vi "Configure Math (Unary Operation).vi"(0 "VISA resource name":refnum<visa-resource-name>, 1 "Enable Math Channel (T:Enable)":bool=TRUE, 2 "# of Averages (16)":i32=16, 3 "FFTWindow (0:Rectangular)":u16(ring) items=["Rectangular", "Hanning", "FlatTop"], 5 "Math Channel (5: Function 1)":i32(ring)=5 items=["Function 1"=5, "Function 2"=6, "Function 3"=7, "Function 4"=8], 7 "Math Operand (1: Channel 1)":i32(ring)=1 items=["Channel 1"=1, "Channel 2"=2, "Channel 3"=3, "Channel 4"=4, "Function 1"=5, "Function 2"=6, "Function 3"=7, "Function 4"=8, "Memory 1"=9, "Memory 2"=10, "Memory 3"=11, "Memory 4"=12], 9 "Math Operation (0: Average)":u16(ring) items=["Average", "Differentiate", "FFT Magnitude", "FFT Phase", "High Pass Filter", "Integrate", "Invert", "Low Pass Filter", "Magnify", "Max", "Min", "Smooth"], 11 "error in (no error)":errorcluster, 12 "Bandwidth (350E6)":dbl=350000000.0, 13 "Smoothing Points (5)":i32=5) -> (4 "VISA resource name out":refnum<visa-resource-name>, 15 "error out":errorcluster)   [LabVIEW 2009, in "Agilent 8000 Series.lvlib"]
doc: "Creates a mathematical expression with one operand."
uses:
  Agilent 8000 Series.lvlib
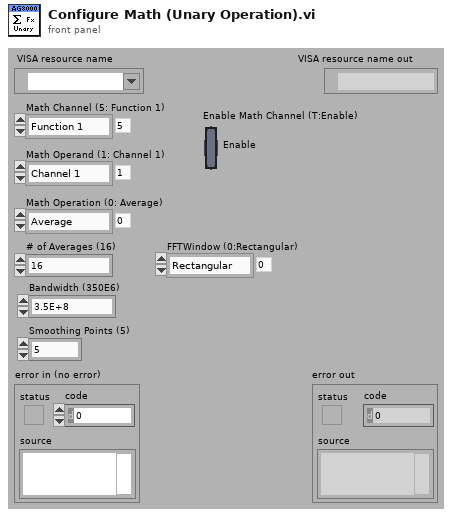
[diagram p1: front panel]
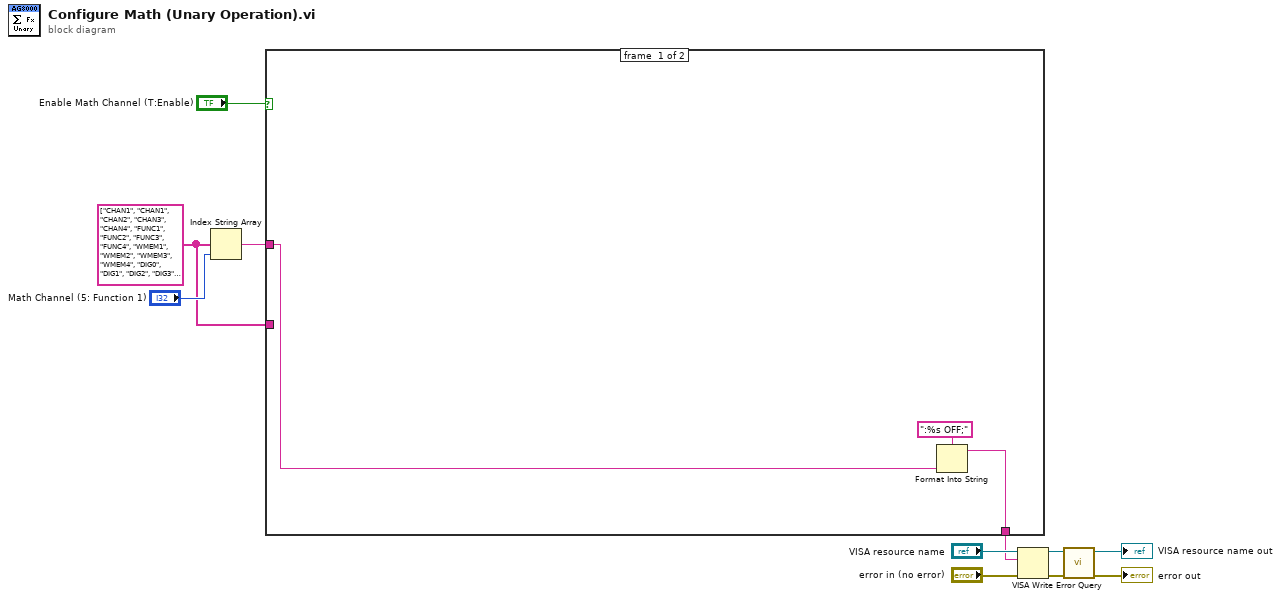
[diagram p0: block diagram]
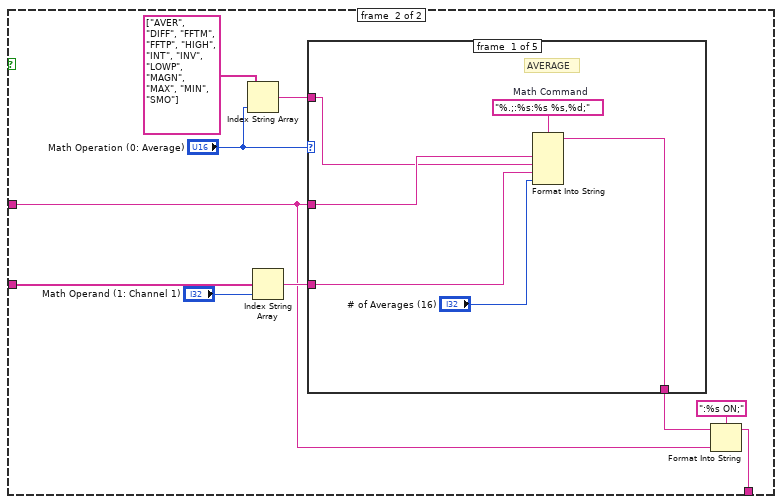
[diagram p2: hidden frame]
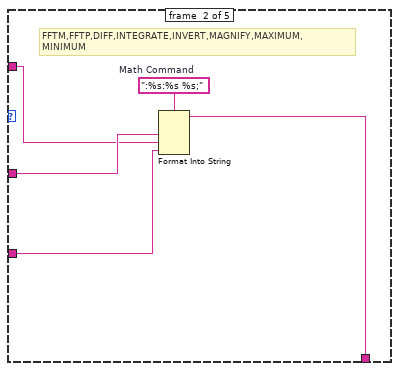
[diagram p3: hidden frame]
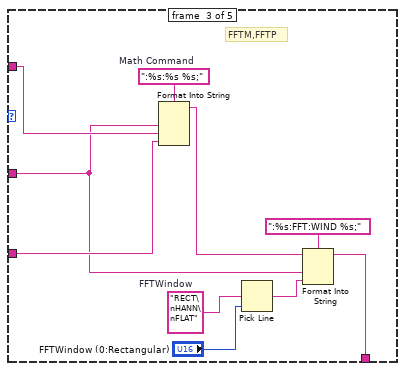
[diagram p4: hidden frame]
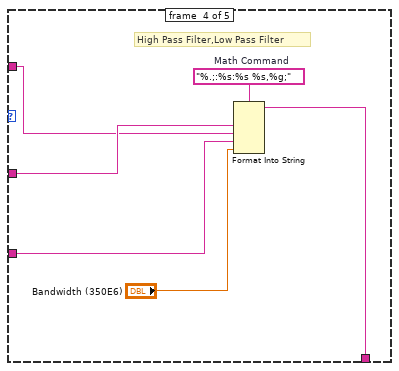
[diagram p5: hidden frame]
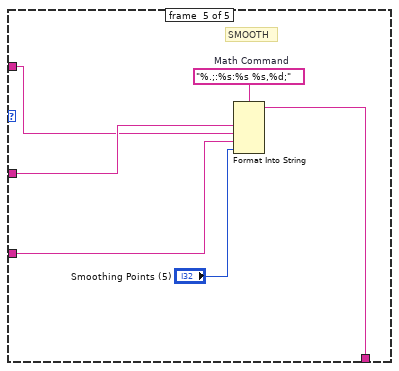
[diagram p6: hidden frame]
diagram:
  w3 = string[] ["CHAN1", "CHAN1", "CHAN2", "CHAN3", "CHAN4", "FUNC1", "FUNC2", "FUNC3", "FUNC4", "WMEM1", "WMEM2", "WMEM3", "WMEM4", "DIG0", "DIG1", "DIG2", "DIG3", "DIG4", "DIG5", "DIG6", "DIG7", "DIG8", "DIG9", "DIG10", "DIG11", "DIG12", "DIG13", "DIG14", "DIG15", "AUX", "LINE"]
  n1 = Index String Array(1:"Math Channel (5: Function 1)", 2:w3) -> (0:w4:string)  [unwired: 1 in]
  n2 = case shown="True" "Enable Math Channel (T:Enable)" {
    tunnel: w4 -> [w13 w16]
    tunnel: w3 -> [_ w20]
    tunnel: [w12 w15] -> w1
    frame #0 {
      n3 = Format Into String(format string=":%s OFF;", w13) -> (resulting string=w12:string)  [unwired: 2 in, 1 out]
    }
    frame #1 {
      n4 = Index String Array(1:"Math Operation (0: Average)", 2:string[] ["AVER", "DIFF", "FFTM", "FFTP", "HIGH", "INT", "INV", "LOWP", "MAGN", "MAX", "MIN", "SMO"]) -> (0:w22:string)  [unwired: 1 in]
      n5 = Index String Array(1:"Math Operand (1: Channel 1)", 2:w20) -> (0:w19:string)  [unwired: 1 in]
      n6 = case shown="11" "Math Operation (0: Average)" {
        tunnel: w16 -> [w30 w35 w37 w51 w57]
        tunnel: w22 -> [w29 w34 w45 w50 w56]
        tunnel: w19 -> [w28 w33 w44 w49 w55]
        tunnel: [w25 w31 w36 w46 w52] -> w18
        frame #0 {
          w27 = "%.;:%s:%s %s,%d;"  # Math Command
          # "AVERAGE"
          n7 = Format Into String(format string=w27, w30, w29, w28, "# of Averages (16)") -> (resulting string=w25:string)  [unwired: 2 in, 1 out]
        }
        frame #1 {
          w32 = ":%s:%s %s;"  # Math Command
          # "FFTM,FFTP,DIFF,INTEGRATE,INVERT,MAGNIFY,MAXIMUM,\nMINIMUM"
          n8 = Format Into String(format string=w32, w35, w34, w33) -> (resulting string=w31:string)  [unwired: 2 in, 1 out]
        }
        frame #2 {
          w42 = "RECT\nHANN\nFLAT"  # FFTWindow
          w43 = ":%s:%s %s;"  # Math Command
          # "FFTM,FFTP"
          n9 = Format Into String(format string=w43, w37, w45, w44) -> (resulting string=w39:string)  [unwired: 2 in, 1 out]
          n10 = Pick Line(multi-line string=w42, line index="FFTWindow (0:Rectangular)") -> (output string=w38:string)  [unwired: 1 in]
          n11 = Format Into String(format string=":%s:FFT:WIND %s;", initial string=w39, w37, w38) -> (resulting string=w36:string)  [unwired: 1 in, 1 out]
        }
        frame #3 {
          w48 = "%.;:%s:%s %s,%g;"  # Math Command
          # "High Pass Filter,Low Pass Filter"
          n12 = Format Into String(format string=w48, w51, w50, w49, "Bandwidth (350E6)") -> (resulting string=w46:string)  [unwired: 2 in, 1 out]
        }
        frame #4 {
          w54 = "%.;:%s:%s %s,%d;"  # Math Command
          # "SMOOTH"
          n13 = Format Into String(format string=w54, w57, w56, w55, "Smoothing Points (5)") -> (resulting string=w52:string)  [unwired: 2 in, 1 out]
        }
      }
      n14 = Format Into String(format string=":%s ON;", initial string=w18, w16) -> (resulting string=w15:string)  [unwired: 1 in, 1 out]
    }
  }
  n15 = VISA Write(VISA resource name="VISA resource name", write buffer=w1, error in (no error)="error in (no error)") -> (VISA resource name out=w7:refnum<visa-resource-name>, error out=w6:errorcluster)  [unwired: 1 out]
  n16 = call "Error Query.vi"("error in (no error)"=w6, "VISA resource name"=w7) -> ("error out"=→"error out":errorcluster, "VISA resource name out"=→"VISA resource name out":refnum<visa-resource-name>)  [unwired: 6 in, 2 out]
